vi "NotifyIcon - Register LabVIEW User Events.vi"(6 "Action":T1, 8 "error in":errorcluster, 10 "Events to register":T2[](array[typedef]), 11 "NotifyIcon reference in":refnum<k24>) -> (0 "error out":errorcluster, 1 "user event - Close application":refnum<user-event>, 2 "Event Registration Refnum":refnum<event-registration>, 3 "NotifyIcon reference out":refnum<k24>)   [LabVIEW 2015]
doc: "Registers a LabVIEW user event to allow the LabVIEW Event Structure to capture events fired from the NotifyIcon.\n\nWire the <b>Event Registration Refnum</b> output to the Dynamic Event Terminal of an Event Structure."
uses:
  System.Windows.Forms
  TypeDefs/NotifyIcon Events.ctl
  TypeDefs/NotifyIcon Event Registration Actions.ctl
  TypeDefs/NotifyIcon User Event Ref.ctl
  TypeDefs/NotifyIcon Event Data.ctl
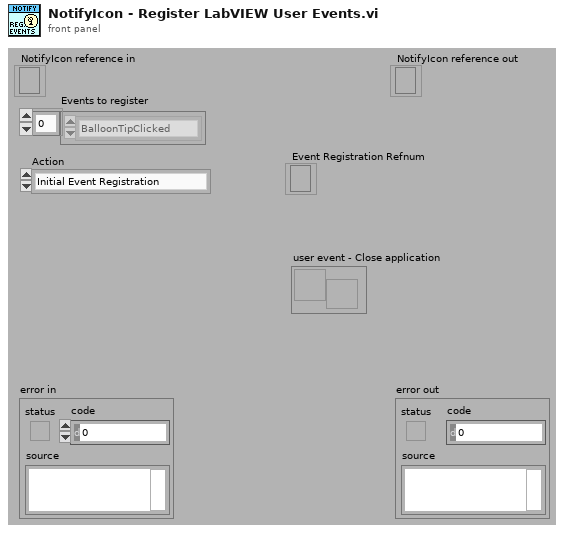
[diagram p1: front panel]
types:
  T1 = typedef "NotifyIcon Event Registration Actions.ctl" = enum16{"Initial Event Registration", "Add to Event Registration", "Destroy Events and Re-register"}
  T2 = typedef "NotifyIcon Events.ctl" = enum16{"BalloonTipClicked", "BalloonTipClosed", "BalloonTipShown", "Click", "Disposed", "DoubleClick", "MouseClick", "MouseDoubleClick", "MouseDown", "MouseMove", "MouseUp", "MenuItemClick", "MenuItemSelect"}
  T3 = typedef "NotifyIcon Event Data.ctl" = cluster{"NotifyIcon Event":T2, "Data String":string}
  T4 = typedef "NotifyIcon User Event Ref.ctl" = refnum<user-event>
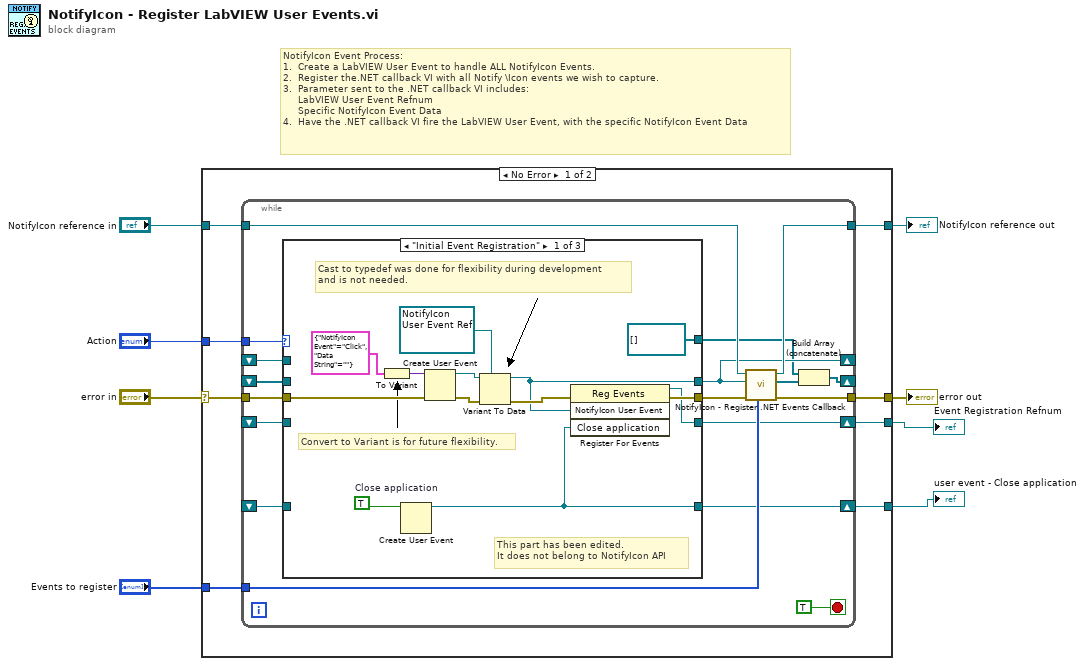
[diagram p0: block diagram]
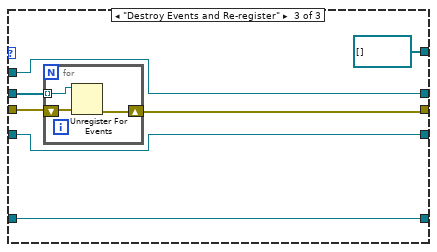
[diagram p3: hidden frame]
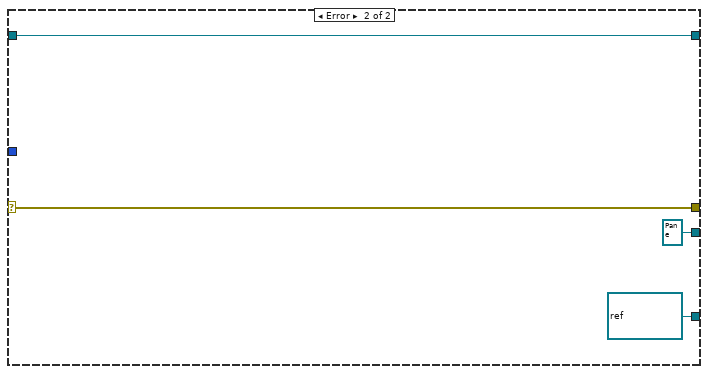
[diagram p4: hidden frame]
diagram:
  # "NotifyIcon Event Process:\n1.  Create a LabVIEW User Event to handle ALL NotifyIcon Events.\n2.  Register the.NET callback VI with all Notify \\Icon events we wish to capture.\n3.  Parameter sent to the .NET callback VI includes:\n     LabVIEW User Event Refnum\n     Specific NotifyIcon Event Data\n4.  Have the .NET callback VI fire the LabVIEW User Event, with the specific NotifyIcon Event Data"
  n1 = case shown="No Error" "error in" {
    selector: "error in" -> [w11 w66]
    tunnel: "NotifyIcon reference in" -> [w16 w65]
    tunnel: "Events to register" -> [w15 _]
    tunnel: [w14 w65] -> w6
    tunnel: [w13 w66] -> w5
    tunnel: [w12 refnum<event-registration> refnum ("Event Registration Refnum")] -> w2
    tunnel: "Action" -> [w10 _]
    tunnel: [w9 refnum<user-event> refnum ("Close application")] -> w1
    frame No Error {
      n2 = while {
        tunnel: w16 -> [w33]
        tunnel: w15 -> [w32]
        tunnel: [w31] -> w14
        tunnel: [w30] -> w13
        tunnel: w11 -> [w28]
        tunnel: w10 -> [w26]
        shift-right: [w25] -> _
        shift-left: _ -> [w24]
        shift-right: [w29] -> w12
        shift-left: _ -> [w23]
        shift-right: [w20] -> _
        shift-left: _ -> [w22]
        shift-right: [w18] -> w9
        shift-left: _ -> [w17]
        stop <- TRUE stop-if-true
        n3 = case shown="\"Initial Event Registration\"" w26 {
          tunnel: [w41 w51 w56] -> w34
          tunnel: [w40 w52 w57] -> w25
          tunnel: [w39 w50 w55] -> w29
          tunnel: w28 -> [w38 w51 w59]
          tunnel: w24 -> [_ w52 w57]
          tunnel: w23 -> [_ w50 w55]
          tunnel: w22 -> [_ w49 w58]
          tunnel: [refnum<k27>[] [] w49 refnum<k27>[] []] -> w19
          tunnel: [w35 w48 w53] -> w18
          tunnel: w17 -> [_ w48 w53]
          frame "Initial Event Registration" {
            w36 = TRUE  # Close application
            # "This part has been edited. \nIt does not belong to NotifyIcon API"
            # "Cast to typedef was done for flexibility during development\nand is not needed."
            # "Convert to Variant is for future flexibility."
            n4 = To Variant(anything=T3 {"NotifyIcon Event"=enum."Click", "Data String"=""} ("NotifyIcon Event Data")) -> (Variant=w45:variant)
            n5 = Create User Event(user event datatype=w36) -> (user event=w35:refnum<user-event>)  [unwired: 1 in, 1 out]
            n6 = Create User Event(user event datatype=w45, error in=w38) -> (user event=w44:refnum<user-event>, error out=w47:errorcluster)
            n7 = Variant To Data(error in=w47, type=T4 refnum ("NotifyIcon User Event"), Variant=w44) -> (data=w40:T4, error out=w46:errorcluster)
            n8 = register-events(error in=w46, w40, w35) -> (reference out=w39:refnum<event-registration>, error out=w41:errorcluster)  [unwired: 1 in]
          }
          frame "Add to Event Registration", Default {
          }
          frame "Destroy Events and Re-register" {
            n9 = for {
              tunnel: w58 -> [w61] mode=indexing
              shift-right: [w60] -> w56
              shift-left: w59 -> [w62]
              n10 = Unregister For Events(event registration refnum=w61, error in=w62) -> (error out=w60:errorcluster)
            }
          }
        }
        n11 = call "NotifyIcon - Register .NET Events Callback.vi"("Events to register"=w32, "error in (no error)"=w34, "NotifyIcon User Event Ref"=w25, "NotifyIcon reference in"=w33) -> ("error out"=w30:errorcluster, ".NET event refs"=w21:refnum<k27>[], "NotifyIcon reference out"=w31:refnum<k24>)  [unwired: 5 in]
        n12 = Build Array (concatenate)(w19, w21) -> (w20:refnum<k27>[])
      }
    }
    frame Error {
    }
  }
  "NotifyIcon reference out" <- w6
  "error out" <- w5
  "Event Registration Refnum" <- w2
  "user event - Close application" <- w1
